vi "String Compare.vi"(1 "String 1":string, 2 "String 2":string, 4 "Case Insensitive? (f)":bool) -> (6 "Equivalent?":bool)   [LabVIEW 2011]
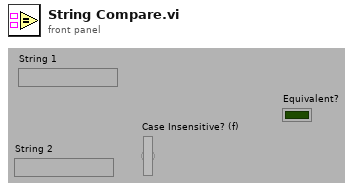
[diagram p1: front panel]
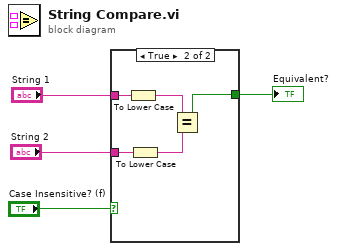
[diagram p0: block diagram]
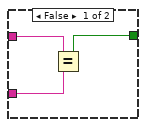
[diagram p2: hidden frame]
diagram:
  n1 = case shown="True" "Case Insensitive? (f)" {
    tunnel: "String 1" -> [w7 w12]
    tunnel: "String 2" -> [w6 w11]
    tunnel: [w5 w8] -> w1
    frame False {
      n2 = Equal?(x=w7, y=w6) -> (x = y?=w5:bool)
    }
    frame True {
      n3 = To Lower Case(string=w12) -> (all lower case string=w10:string)
      n4 = To Lower Case(string=w11) -> (all lower case string=w9:string)
      n5 = Equal?(x=w10, y=w9) -> (x = y?=w8:bool)
    }
  }
  "Equivalent?" <- w1
